vi "parse pixie data.vi"(8 "error in (no error)":errorcluster, 9 "scale factor":u32=10, 10 "Pixie input array 2":u16[](array[numeric])=array[250000 elements], 11 "Pixie input array":u16[](array[numeric])=array[250000 elements]) -> (0 "error out":errorcluster, 2 "time 0-3":u32[][](array[numeric]), 3 "Pixie output array":u32[](array[numeric]), 5 "0-3 events":dbl[][](array[numeric]), 6 "Sum of gated counts":i32=2628)   [LabVIEW 2016]
doc: "Using c code, This vi takes the hard gate limits and determines if each value in the pixie input array passes test"
uses:
  Drivers/Pixie4DLL.dll
panel:
  out "number of events":dbl=2717.0
  out "channel 0":u16[](array[numeric])
  out "size of pixie array":u32=28932
  out "Channel 3":i32[](array[numeric])
  out "Channel 2":i32[](array[numeric])
  out "Channel 1":i32[](array[numeric])
  out "Channel 0":i32[](array[numeric])
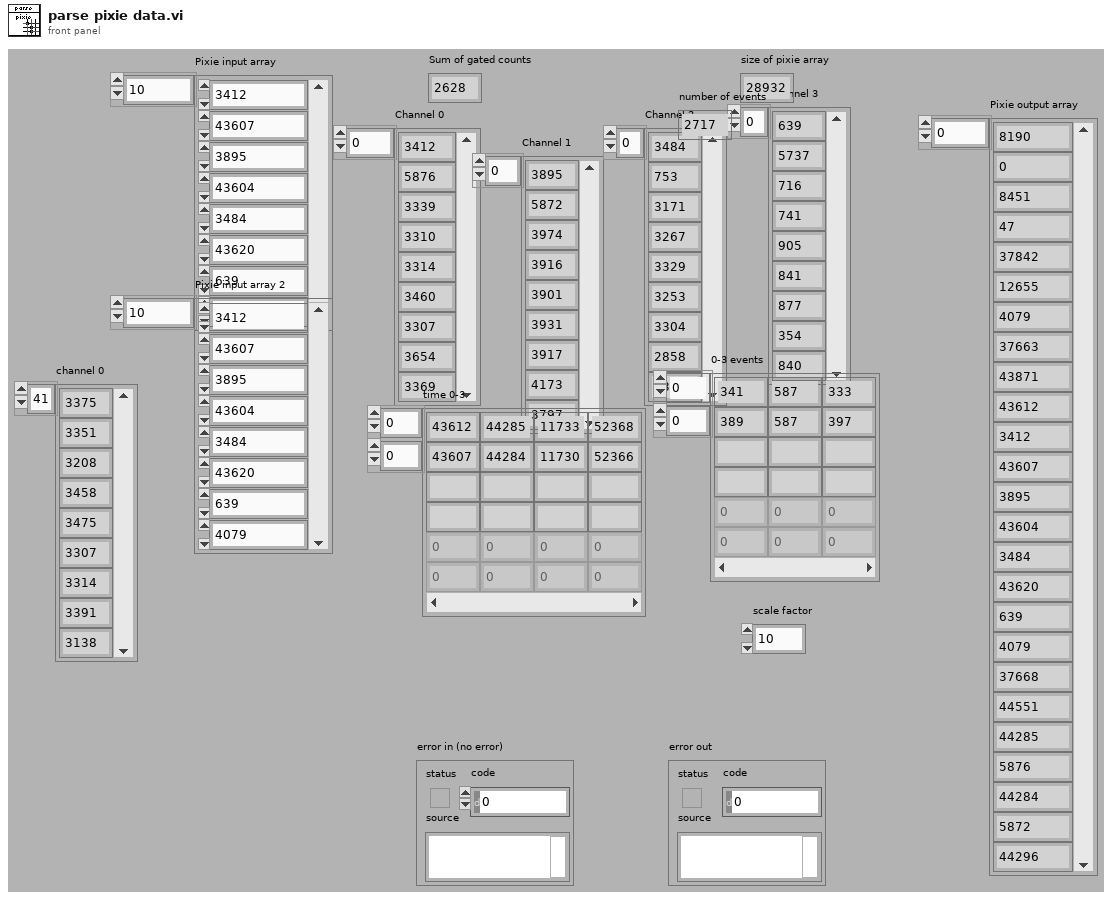
[diagram p1: front panel]
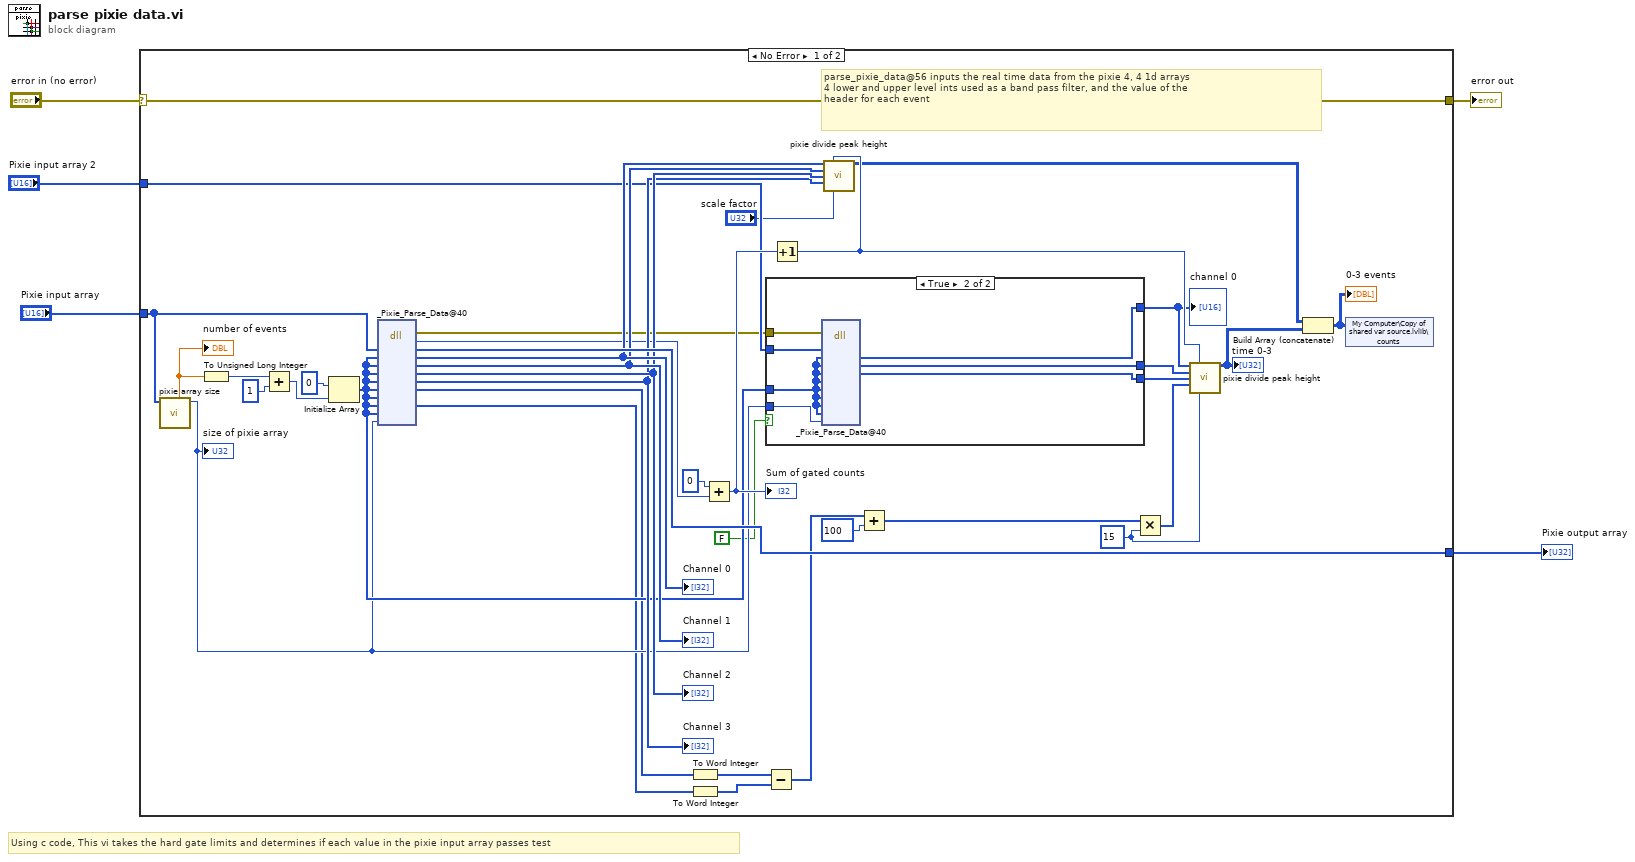
[diagram p0: block diagram]
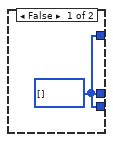
[diagram p2: hidden frame]
diagram:
  # "Using c code, This vi takes the hard gate limits and determines if each value in the pixie input array passes test"
  n1 = case shown="No Error" "error in (no error)" {
    selector: "error in (no error)" -> [w41 w51]
    tunnel: "Pixie input array" -> [w31 w52]
    tunnel: [w42 w52] -> w4
    tunnel: [w41 w51] -> w2
    tunnel: "Pixie input array 2" -> [w25 _]
    frame No Error {
      w8 = u32 15 ("scale factor")
      # "parse_pixie_data@56 inputs the real time data from the pixie 4, 4 1d arrays\n4 lower and upper level ints used as a band pass filter, and the value of the\nheader for each event"
      n2 = call "pixie array size.vi"("Pixie input array"=w31) -> ("size of pixie array"=w26:u32, "number of events"=w30:dbl)  [unwired: 6 in, 3 out]
      "size of pixie array" <- w26
      "number of events" <- w30
      n3 = To Unsigned Long Integer(number=w30) -> (unsigned 32bit integer=w28:u32)
      n4 = Add(x=w28, y=1) -> (x+y=w29:u32)
      n5 = Initialize Array(u32 0 ("element"), w29) -> (w27:u32[])
      n6 = dll-call lib="D:/Users/wymanm/Desktop/DAQuiri - 2017a/PRIME DAQ 2017a/Drivers/Pixie4DLL.dll" fn="_Pixie_Parse_Data@40"("listmodedata"=w31, "channel 0"=w27, "channel 1"=w27, "channel 2"=w27, "channel 3"=w27, "Time 0"=w27, "Time 1"=w27, "Time 2"=w27, "Time 3"=w27, "size"=w26) -> (error out=w24:errorcluster, "return type"=w32:i16, "listmodedata"=w42:u16[], "channel 0"=w40:u16[], "channel 1"=w39:u16[], "channel 2"=w38:u16[], "channel 3"=w37:u16[], "Time 0"=w12:u16[], "Time 2"=w10:u16[])  [unwired: 3 in, 4 out]
      "Channel 0" <- w40
      "Channel 1" <- w39
      "Channel 2" <- w38
      "Channel 3" <- w37
      n7 = To Word Integer(number=w12) -> (16bit integer=w11:i16[])
      n8 = To Word Integer(number=w10) -> (16bit integer=w9:i16[])
      n9 = Add(x=u16 0, y=w32) -> (x+y=w35:u16)
      "Sum of gated counts" <- w35
      n10 = case shown="True" FALSE {
        tunnel: w27 -> [_ w50]
        tunnel: w26 -> [_ w49]
        tunnel: w25 -> [_ w48]
        tunnel: w24 -> [_ w47]
        tunnel: [w43 w46] -> w22
        tunnel: [w43 w45] -> w17
        tunnel: [w43 w44] -> w13
        frame False {
          w43 = u16[] [] ("channel 0")
        }
        frame True {
          n11 = dll-call lib="D:/Users/wymanm/Desktop/DAQuiri - 2017a/PRIME DAQ 2017a/Drivers/Pixie4DLL.dll" fn="_Pixie_Parse_Data@40"(error in=w47, "listmodedata"=w48, "channel 0"=w50, "channel 1"=w50, "channel 2"=w50, "channel 3"=w50, "Time 0"=w50, "Time 1"=w50, "Time 2"=w50, "Time 3"=w50, "size"=w49) -> ("channel 0"=w44:u16[], "channel 1"=w46:u16[], "channel 2"=w45:u16[])  [unwired: 2 in, 10 out]
        }
      }
      "channel 0" <- w13
      n12 = Subtract(x=w11, y=w9) -> (x-y=w19:i16[])
      n13 = Increment(x=w35) -> (x+1=w23:u16)
      n14 = call "pixie divide peak height.vi"("channel 0"=w40, "size of array"=w23, "channel 1"=w39, "channel 2"=w38, "channel 3"=w37, "scale factor"="scale factor") -> ("output channel 0-3"=w21:u32[][])  [unwired: 8 in, 1 out]
      n15 = Add(x=w19, y=i16 100) -> (x+y=w16:i16[])
      n16 = Multiply(x=w16, y=w8) -> (x*y=w14:u32[])
      n17 = call "pixie divide peak height.vi"("channel 0"=w13, "size of array"=w23, "channel 1"=w22, "channel 2"=w17, "channel 3"=w14, "scale factor"=w8) -> ("output channel 0-3"=w20:u32[][])  [unwired: 8 in, 1 out]
      "time 0-3" <- w20
      n18 = Build Array (concatenate)(w21, w20) -> (w6:u32[][])
      "0-3 events" <- w6
      n19 = shared-variable "My Computer\\Copy of shared var source.lvlib\\counts"(w6) -> ()  [unwired: 1 in, 1 out]
    }
    frame Error {
    }
  }
  "Pixie output array" <- w4
  "error out" <- w2
